vi "Shutdown.vi"(8 "error in":errorcluster, 11 "Modbus instance in":refnum<class "Modbus API.lvclass">) -> (0 "error out":errorcluster)   [LabVIEW 2013, in "Modbus Library - Advance.lvlib" / "Modbus API.lvclass"]
doc: "Performs any actions needed to shutdown and clean up the Modbus instance provided."
uses:
  Modbus API.lvclass
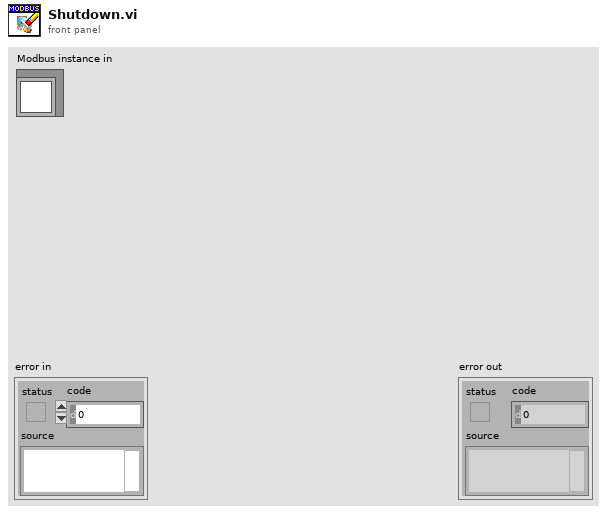
[diagram p1: front panel]
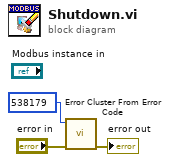
[diagram p0: block diagram]
diagram:
  n1 = call <vilib>:"Error Cluster From Error Code.vi"("error in (no error)"="error in", "error code (0)"=538179) -> ("error out"=→"error out":errorcluster)  [unwired: 7 in]
